vi "Init.vi"(3 "Container State":T3, 4 "Previous State":variant, 5 "Previous Version":T2) -> (2 "Current State":T1)   [LabVIEW 2016, in "MGI Path Selector.xctl"]
uses:
  <userlib>/_MGI/User Interface/Path Selector XControl/MGI Path Selector.xctl
  <userlib>/_MGI/User Interface/Path Selector XControl/State.ctl
  <userlib>/_MGI/User Interface/Path Selector XControl/Class Hierarchy/MGI Path Selector.lvclass
  <vilib>/_xctls/Container State.ctl
  <vilib>/_xctls/Version.ctl
  <userlib>/_MGI/User Interface/Path Selector XControl/Class Hierarchy/Persistent Path Selector/MGI Persistent Path Selector.lvclass
  C:/Program Files (x86)/National Instruments/LabVIEW 2016/user.lib/_MGI/User Interface/Path Selector XControl/Class Hierarchy/MGI Path Selector.lvclass
  <vilib>/_xctls/XControlSupport.lvlib
panel:
  in  "Default Indicator State":T1
  in  "Default Control State":T1
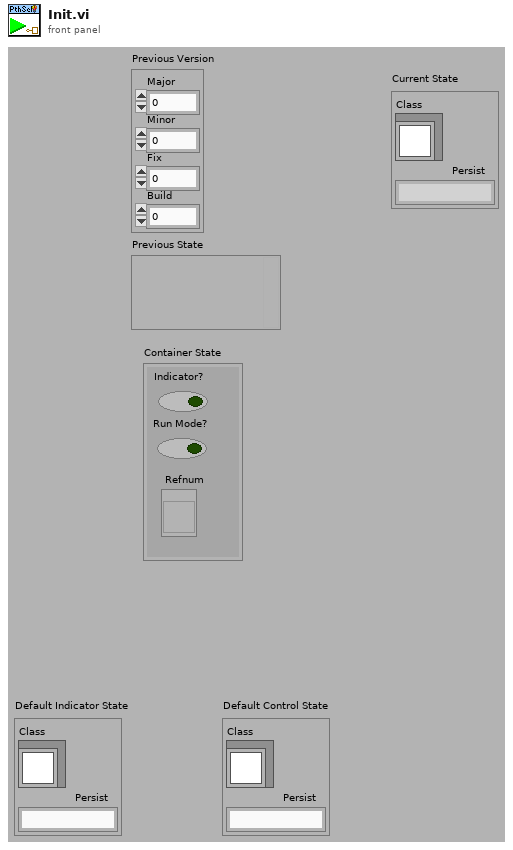
[diagram p1: front panel]
types:
  T1 = typedef "MGI Path Selector.xctl/State.ctl" = cluster{"Class":refnum<class "MGI Path Selector.lvclass">, "Persist":string}
  T2 = typedef "XControlSupport.lvlib/Version.ctl" = cluster{"Major":u16, "Minor":u16, "Fix":u16, "Build":u16}
  T3 = typedef "XControlSupport.lvlib/Container State.ctl" = cluster{"Indicator?":bool, "Run Mode?":bool, " Refnum":refnum<vi>}
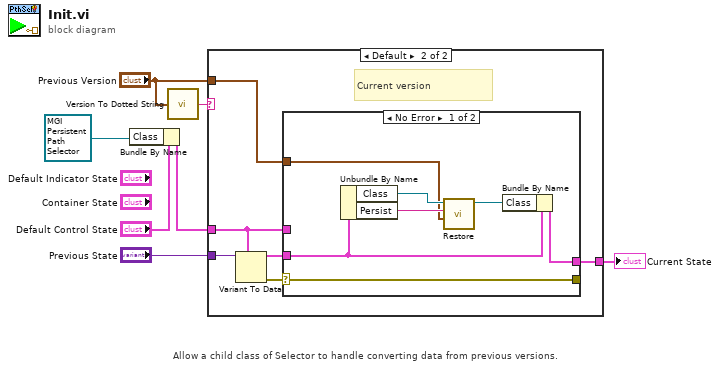
[diagram p0: block diagram]
diagram:
  # "Allow a child class of Selector to handle converting data from previous versions."
  n1 = Bundle By Name(cluster="Default Control State", "Class"=refnum<class "MGI Persistent Path Selector.lvclass"> refnum ("Persistent Path Selector.lvclass")) -> (w3:T1)
  n2 = call <vilib>:"Version To Dotted String.vi"("Version"="Previous Version") -> ("String Version"=w6:string)
  n3 = case shown="Default" w6 {
    tunnel: "Previous State" -> [_ w14]
    tunnel: [w8 w11] -> w5
    tunnel: w3 -> [w8 w9]
    tunnel: "Previous Version" -> [_ w10]
    frame "0.0.0.0" {
    }
    frame Default {
      # "Current version"
      n4 = Variant To Data(type=w9, Variant=w14) -> (data=w12:T1, error out=w13:errorcluster)  [unwired: 1 in]
      n5 = case shown="No Error" w13 {
        selector: w13 -> [w21 w22]
        tunnel: w12 -> [w20 _]
        tunnel: [w17 w23] -> w11
        tunnel: w9 -> [_ w23]
        tunnel: [w21 w22] -> _
        tunnel: w10 -> [w15 _]
        frame No Error {
          n6 = Unbundle By Name(w20) -> ("Class"=w19:refnum<class "MGI Path Selector.lvclass">, "Persist"=w16:string)
          n7 = call-dynamic "Restore.vi"("Previous Version"=w15, "Data"=w16, "Path Selector in"=w19) -> ("Path Selector out"=w18:refnum<class "MGI Path Selector.lvclass">)  [unwired: 7 in, 1 out]
          n8 = Bundle By Name(cluster=w20, "Class"=w18) -> (w17:T1)
        }
        frame Error {
          # "Error converting previously \nsaved state. Use default instead."
        }
      }
    }
  }
  "Current State" <- w5
